vi "svfa_Zoom Configurator.vi"(1 "restart averaging (F)":bool, 5 "fs":dbl format="%.2f", 9 "zoom settings":T1={"frequency range"={"start frequency"=20.0, "stop frequency"=20000.0}, "window"=1, "# of lines"=0, "% overlap"=0.0} {"% overlap" format="%.2f"; "window" items=["None ", "Hanning", "Hamming", "Blackman-Harris", "Exact Blackman", "Blackman", "Flat Top", "4 Term B-Harris ", "7 Term B-Harris", "Low Sidelobe", "Force - Exponential"]; "frequency range"."stop frequency" format="%.2f"; "frequency range"."start frequency" format="%.2f"}, 11 "error in (no error)":errorcluster) -> (6 "fs":dbl format="%.2f", 8 "Max Block Size":i32, 10 "zoom FFT settings":T2={"zoom settings"={"center frequency"=-inf, "zoom"=1, "trim"=1.0}, "FFT settings"={"window"=enum."Hanning", "window size"=-1, "FFT size"=1024, "%overlap"=0.0}} {"FFT settings"."%overlap" min=0.0 max=100.0 format="%.2f"; "zoom settings"."trim" min=1.0 format="%.2f"; "zoom settings"."center frequency" format="%.2f"; "zoom settings"."zoom" min=1}, 15 "error out":errorcluster)   [LabVIEW 2017]
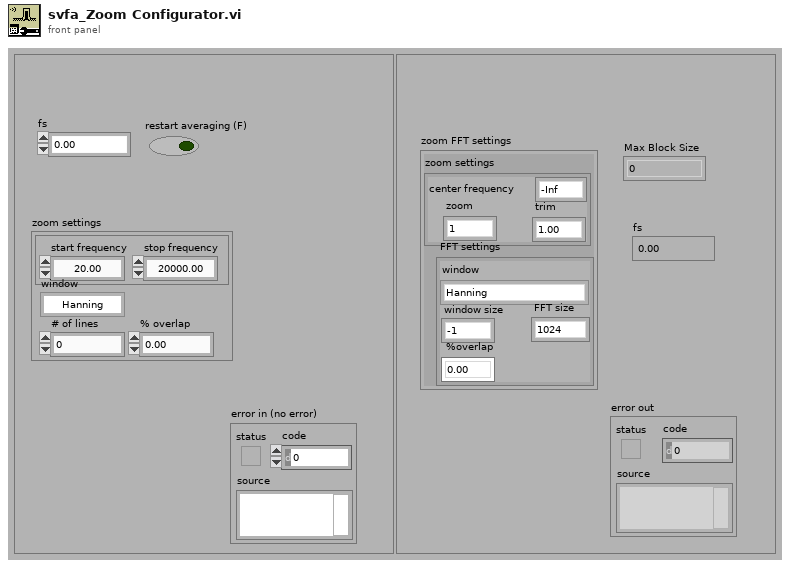
[diagram p1: front panel]
types:
  T1 = cluster{"frequency range":cluster{"start frequency":dbl, "stop frequency":dbl}, "window":u16, "# of lines":i32, "% overlap":dbl}
  T2 = cluster{"zoom settings":cluster{"center frequency":dbl, "zoom":i32, "trim":dbl}, "FFT settings":cluster{"window":enum16{"None ", "Hanning", "Hamming", "Blackman-Harris", "Exact Blackman", "Blackman", "Flat Top", "4 Term B-Harris ", "7 Term B-Harris", "Low Sidelobe"}, "window size":i32, "FFT size":i32, "%overlap":dbl}}
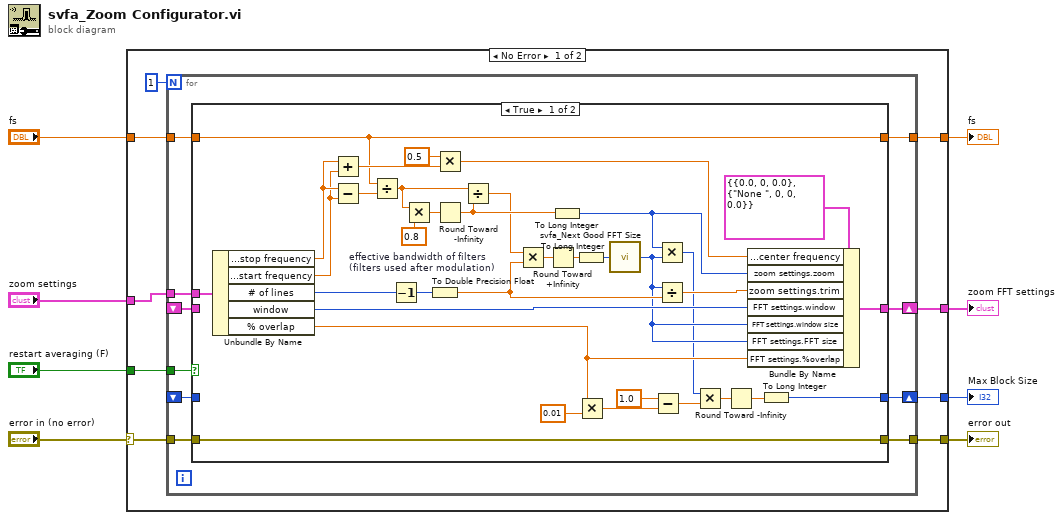
[diagram p0: block diagram]
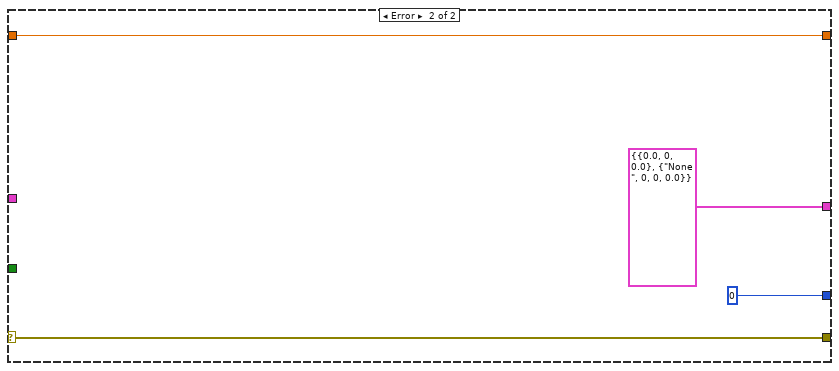
[diagram p3: hidden frame]
diagram:
  n1 = case shown="No Error" "error in (no error)" {
    selector: "error in (no error)" -> [w15 w70]
    tunnel: "zoom settings" -> [w17 _]
    tunnel: [w16 w70] -> w7
    tunnel: [w11 w67] -> w6
    tunnel: [w10 0] -> w5
    tunnel: [w13 T2 {"zoom settings"={"center frequency"=0.0, "zoom"=0, "trim"=0.0}, "FFT settings"={"window"=enum."None ", "window size"=0, "FFT size"=0, "%overlap"=0.0}} ("zoom FFT settings (dupl)")] -> w4
    tunnel: "fs" -> [w12 w67]
    tunnel: "restart averaging (F)" -> [w14 _]
    frame No Error {
      n2 = for {
        N: 1 -> [_]
        shift-left: _ -> [w18]
        shift-right: [w19] -> w10
        tunnel: [w20] -> w11
        tunnel: w14 -> [w23]
        shift-left: _ -> [w21]
        shift-right: [w22] -> w13
        tunnel: w12 -> [w24]
        tunnel: w15 -> [w25]
        tunnel: [w26] -> w16
        tunnel: w17 -> [w27]
        n3 = case shown="True" w23 {
          tunnel: w27 -> [w62 _]
          tunnel: [w30 w65] -> w26
          tunnel: [w61 w63] -> w19
          tunnel: w25 -> [w30 w65]
          tunnel: [w52 w66] -> w22
          tunnel: w24 -> [w28 w64]
          tunnel: w21 -> [_ w66]
          tunnel: [w28 w64] -> w20
          tunnel: w18 -> [_ w63]
          frame True {
            w41 = 0.8  # effective bandwidth of filters (filters used after modulation)
            n4 = Unbundle By Name(w62) -> ("frequency range.stop frequency"=w32:dbl, "frequency range.start frequency"=w31:dbl, "# of lines"=w33:i32, "window"=w60:u16, "% overlap"=w53:dbl)
            n5 = Add(x=w32, y=w31) -> (x+y=w49:dbl)
            n6 = Subtract(x=w32, y=w31) -> (x-y=w48:dbl)
            n7 = Divide(x=w28, y=w48) -> (x/y=w42:dbl)
            n8 = Decrement(x=w33) -> (x-1=w39:i32)
            n9 = Multiply(x=w42, y=w41) -> (x*y=w47:dbl)
            n10 = To Double Precision Float(number=w39) -> (double precision float=w38:dbl)
            n11 = Multiply(x=0.5 ("y"), y=w49) -> (x*y=w37:dbl)
            n12 = Round Toward -Infinity ("Round To -Infinity")(1:w47) -> (0:w43:dbl)
            n13 = Divide(x=w42, y=w43) -> (x/y=w40:dbl)
            n14 = Multiply(x=w40, y=w38) -> (x*y=w46:dbl)
            n15 = Round Toward +Infinity ("Round To +Infinity")(x=w46) -> (ceil(x): smallest int >= x=w45:dbl)
            n16 = To Long Integer(number=w43) -> (32bit integer=w36:i32)
            n17 = To Long Integer(number=w45) -> (32bit integer=w44:i32)
            n18 = Multiply(x=w53, y=0.01) -> (x*y=w57:dbl)
            n19 = call <vilib>:"svfa_Next Good FFT Size.vi"("FFT Size"=w44) -> ("least bigger good size"=w34:i32)
            n20 = Subtract(x=1.0, y=w57) -> (x-y=w56:dbl)
            n21 = Multiply(x=w36, y=w34) -> (x*y=w29:i32)
            n22 = Divide(x=w34, y=w38) -> (x/y=w35:dbl)
            n23 = Multiply(x=w29, y=w56) -> (x*y=w54:dbl)
            n24 = Round Toward -Infinity ("Round To -Infinity")(1:w54) -> (0:w55:dbl)
            n25 = Bundle By Name(cluster=T2 {"zoom settings"={"center frequency"=0.0, "zoom"=0, "trim"=0.0}, "FFT settings"={"window"=enum."None ", "window size"=0, "FFT size"=0, "%overlap"=0.0}} ("Output Cluster"), "zoom settings.center frequency"=w37, "zoom settings.zoom"=w36, "zoom settings.trim"=w35, "FFT settings.window"=w60, "FFT settings.window size"=w34, "FFT settings.FFT size"=w34, "FFT settings.%overlap"=w53) -> (w52:T2)
            n26 = To Long Integer(number=w55) -> (32bit integer=w61:i32)
          }
          frame False {
          }
        }
      }
    }
    frame Error {
    }
  }
  "zoom FFT settings" <- w4
  "error out" <- w7
  "fs" <- w6
  "Max Block Size" <- w5
